vi "load from file and run all.vi"(8 "error in":errorcluster, 9 "target alias":string, 10 "tokenized path":T1, 11 "message queue in":T2) -> (0 "error out":errorcluster, 3 "message queue out":T2)   [LabVIEW 2013, in "TBD execution service.lvlib"]
doc: "This VI uses the 'tokenized path' and 'target alias' inputs to load and run the specified target configuration within that file. \n\nUse the 'Path to Array of Strings' to convert the configuration file's path location into the format that is required by the 'tokenized path' input. This conversion is required so that the file path can be platform agnostic."
uses:
  TBD execution service.lvlib
  <vilib>/NI/AMC/Message Queue.ctl
  <vilib>/NI/AMC/Message.ctl
  <vilib>/NI/Tools/Keyed Array/KeyedArray.ctl
  tokenized path.ctl
  command commands to rtexe process.ctl
  <vilib>/NI/Tools/Keyed Array/Tools_KeyedArray.lvlib
  <vilib>/NI/AMC/AMC.lvlib
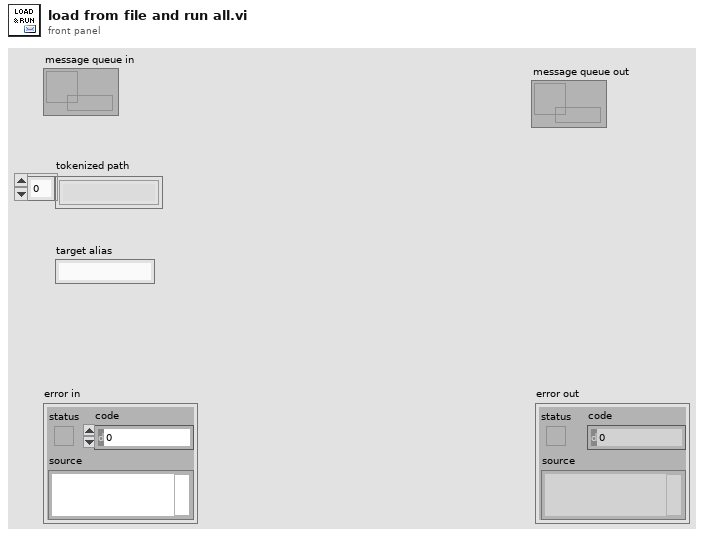
[diagram p1: front panel]
types:
  T1 = typedef "TBD execution service.lvlib/tokenized path.ctl" = string[]
  T2 = typedef "AMC.lvlib/Message Queue.ctl" = refnum<queue>
  T3 = typedef "TBD execution service.lvlib/command commands to rtexe process.ctl" = enum16{"Initialize", "Add Search Paths", "Load from File", "Unload File", "Open All Engines", "Open Single Engine", "Initialize All Engines", "Initialize Single Engine", "Start All", "Start Single", "Pause All", "Pause Single", "Stop All", "Stop Single", "Close All", "Close Single", "Set Safe State All", "Set Safe State Single", "Get Status", "Exit", "Error", "Load Bitfile", "Unload Bitfile", "Clear Faults Single", "Clear Faults All"}
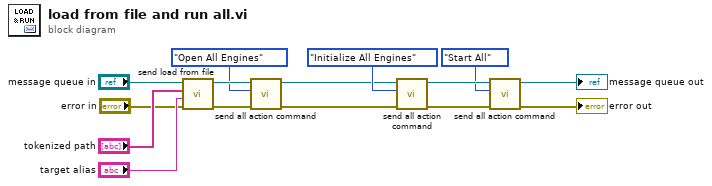
[diagram p0: block diagram]
diagram:
  n1 = call "send load from file.vi"("error in"="error in", "target alias"="target alias", "tokenized path"="tokenized path", "message queue in"="message queue in") -> ("error out"=w13:errorcluster, "message queue out"=w12:T2)  [unwired: 6 in]
  n2 = call "send all action command.vi"("error in"=w13, "commands"=command_commands_to_rtexe_process."Open All Engines", "message queue in"=w12) -> ("error out"=w4:errorcluster, "message queue out"=w3:T2)  [unwired: 7 in]
  n3 = call "send all action command.vi"("error in"=w4, "commands"=command_commands_to_rtexe_process."Initialize All Engines", "message queue in"=w3) -> ("error out"=w15:errorcluster, "message queue out"=w14:T2)  [unwired: 7 in]
  n4 = call "send all action command.vi"("error in"=w15, "commands"=command_commands_to_rtexe_process."Start All", "message queue in"=w14) -> ("error out"=→"error out":errorcluster, "message queue out"=→"message queue out":T2)  [unwired: 7 in]
